vi "Key Scan Converter.vi"(5 "Input Scancode":i16, 6 "Input Key":string="nul") -> (1 "Scancode -> Key":string, 2 "Key -> Scancode":i16)   [LabVIEW 2017]
doc: "Converts back and forth between Keyboard Keys and Keyboard Decimal values. Automatically handles either Mac or PC. For ease of use with Event Structures."
panel:
  out "Scancodes":i32[](array[numeric])
  out "Keys":string[](array[string])
  in  "Scancode Table":string[][](array[string])=[["ID", "Key", "PC-HEX", "PC-DEC", "MAC-DEC", ""], ["1", "ESC", "1", "1", "53", ""], ["2", "1", "2", "2", "18", ""], ["3", "2", "3", "3", "19", ""], ["4", "3", "4", "4", "20", ""], ["5", "4", "5", "5", "21", ""], ["6", "5", "6", "6", "23", ""], ["7", "6", "7", "7", "22", ""], ["8", "7", "8", "8", "26", ""], ["9", "8", "9", "9", "28", ""], ["10", "9", "0A", "10", "25", ""], ["11", "0", "0B", "11", "29", ""], ["12", "-", "0C", "12", "27", ""], ["13", "=", "0D", "13", "24", ""], ["14", "BKSP", "0E", "14", "51", ""], ["15", "Tab", "0F", "15", "48", ""], ["16", "Q", "10", "16", "12", ""], ["17", "W", "11", "17", "13", ""], ["18", "E", "12", "18", "14", ""], ["19", "R", "13", "19", "15", ""], ["20", "T", "14", "20", "17", ""], ["21", "Y", "15", "21", "16", ""], ["22", "U", "16", "22", "32", ""], ["23", "I", "17", "23", "34", ""], ["24", "O", "18", "24", "31", ""], ["25", "P", "19", "25", "35", ""], ["26", "[", "1A", "26", "33", ""], ["27", "]", "1B", "27", "30", ""], ["28", "Enter", "1C", "28", "36", ""], ["29", "Ctrl", "1D", "29", "59", ""], ["30", "A", "1E", "30", "0", ""], ["31", "S", "1F", "31", "1", ""], ["32", "D", "20", "32", "2", ""], ["33", "F", "21", "33", "3", ""], ["34", "G", "22", "34", "5", ""], ["35", "H", "23", "35", "4", ""], ["36", "J", "24", "36", "38", ""], ["37", "K", "25", "37", "40", ""], ["38", "L", "26", "38", "37", ""], ["39", ";", "27", "39", "41", ""], ["40", "", "28", "40", "", ""], ["41", "`", "29", "41", "", ""], ["42", "L SH", "2A", "42", "", ""], ["43", "\\", "2B", "43", "", ""], ["44", "Z", "2C", "44", "6", ""], ["45", "X", "2D", "45", "7", ""], ["46", "C", "2E", "46", "8", ""], ["47", "V", "2F", "47", "9", ""], ["48", "B", "30", "48", "11", ""], ["49", "N", "31", "49", "45", ""], ["50", "M", "32", "50", "46", ""], ["51", "\"", "\"", "33", "51", ""], ["52", ".", "34", "52", "", ""], ["53", "/", "35", "53", "", ""], ["54", "R SH", "36", "54", "", ""], ["55", "PrintScreen", "37", "55", "", ""], ["56", "Alt", "38", "56", "", ""], ["57", "Space", "39", "57", "49", ""], ["58", "CpsLk", "3A", "58", "", ""], ["59", "F1", "3B", "59", "", ""], ["60", "F2", "3C", "60", "", ""], ["61", "F3", "3D", "61", "", ""], ["62", "F4", "3E", "62", "", ""], ["63", "F5", "3F", "63", "", ""], ["64", "F6", "40", "64", "", ""], ["65", "F7", "41", "65", "", ""], ["66", "F8", "42", "66", "", ""], ["67", "F9", "43", "67", "", ""], ["68", "F10", "44", "68", "", ""], ["69", "Num Lk", "45", "69", "", ""], ["70", "Scrl Lk", "46", "70", "", ""], ["71", "Home", "47", "71", "", ""], ["72", "Up Arrow", "48", "72", "126", ""], ["73", "Pg Up", "49", "73", "", ""], ["74", "- (num)", "4A", "74", "", ""], ["75", "Left Arrow", "4B", "75", "123", ""], ["76", "5 (num) ", "4C", "76", "", ""], ["77", "Right Arrow", "4D", "77", "124", ""], ["78", "+ (num)", "4E", "78", "", ""], ["79", "1 End", "4F", "79", "", ""], ["80", "Down Arrow", "50", "80", "125", ""], ["81", "3 Pg Dn", "51", "81", "", ""], ["82", "0 Ins", "52", "82", "", ""], ["83", "Del", "53", "83", "117", ""], ["84", "SH F1", "54", "84", "", ""], ["85", "SH F2", "55", "85", "", ""], ["86", "SH F3", "56", "86", "", ""], ["87", "SH F4", "57", "87", "", ""], ["88", "SH F5", "58", "88", "", ""], ["89", "SH F6", "59", "89", "", ""], ["90", "SH F7", "5A", "90", "", ""], ["91", "SH F8", "5B", "91", "", ""], ["92", "SH F9", "5C", "92", "", ""], ["93", "SH F10", "5D", "93", "", ""], ["94", "Ctrl F1", "5E", "94", "", ""], ["95", "Ctrl F2", "5F", "95", "", ""], ["96", "Ctrl F3", "60", "96", "", ""], ["97", "Ctrl F4", "61", "97", "", ""], ["98", "Ctrl F5", "62", "98", "", ""], ["99", "Ctrl F6", "63", "99", "", ""], ["100", "Ctrl F7", "64", "100", "", ""], ["101", "Ctrl F8", "65", "101", "", ""], ["102", "Ctrl F9", "66", "102", "", ""], ["103", "Ctrl F10", "67", "103", "", ""], ["104", "Alt F1", "68", "104", "", ""], ["105", "Alt F2", "69", "105", "", ""], ["106", "Alt F3", "6A", "106", "", ""], ["107", "Alt F4", "6B", "107", "", ""], ["108", "Alt F5", "6C", "108", "", ""], ["109", "Alt F6", "6D", "109", "", ""], ["110", "Alt F7", "6E", "110", "", ""], ["111", "Alt F8", "6F", "111", "", ""], ["112", "Alt F9", "70", "112", "", ""], ["113", "Alt F10", "71", "113", "", ""], ["114", "Ctrl PtScr", "72", "114", "", ""], ["115", "Ctrl L Arrow", "73", "115", "", ""], ["116", "Ctrl R Arrow", "74", "116", "", ""], ["117", "Ctrl End", "75", "117", "", ""], ["118", "Ctrl PgDn", "76", "118", "", ""], ["119", "Ctrl Home", "77", "119", "", ""], ["120", "Alt 1", "78", "120", "", ""], ["121", "Alt 2", "79", "121", "", ""], ["122", "Alt 3", "7A", "122", "", ""], ["123", "Alt 4", "7B", "123", "", ""], ["124", "Alt 5", "7C", "124", "", ""], ["125", "Alt 6", "7D", "125", "", ""], ["126", "Alt 7", "7E", "126", "", ""], ["127", "Alt 8", "7F", "127", "", ""], ["128", "Alt 9", "80", "128", "", ""], ["129", "Alt 0", "81", "129", "", ""], ["130", "Alt - ", "82", "130", "", ""], ["131", "Alt =", "82", "130", "", ""], ["132", "Ctrl PgUp", "84", "132", "", ""], ["133", "F11", "85", "133", "", ""], ["134", "F12", "86", "134", "", ""], ["135", "SH F11", "87", "135", "", ""], ["136", "SH F12", "88", "136", "", ""], ["137", "Ctrl F11", "89", "137", "", ""], ["138", "Ctrl F12", "8A", "138", "", ""], ["139", "Alt F11", "8B", "139", "", ""], ["140", "Alt F12", "8C", "140", "", ""], ["141", "Ctrl Up Arrow", "8C", "140", "", ""], ["142", "Ctrl - (num)", "8E", "142", "", ""], ["143", "Ctrl 5 (num)", "8F", "143", "", ""], ["144", "Ctrl + (num)", "90", "144", "", ""], ["145", "Ctrl Dn  Arrow", "91", "145", "", ""], ["146", "Ctrl Ins", "92", "146", "", ""], ["147", "Ctrl Del", "93", "147", "", ""], ["148", "Ctrl Tab", "94", "148", "", ""], ["149", "Ctrl / (num)", "95", "149", "", ""], ["150", "Ctrl * (num)", "96", "150", "", ""], ["151", "Alt Home", "97", "151", "", ""], ["152", "Alt Up Arrow", "98", "152", "", ""], ["153", "Alt PgUp", "99", "153", "", ""], ["154", "", "9A", "154", "", ""], ["155", "Alt Left Arrow", "9B", "155", "", ""], ["156", "", "9C", "156", "", ""], ["157", "Alt Rt Arrow", "9D", "157", "", ""], ["158", "", "9E", "158", "", ""], ["159", "Alt End", "9F", "159", "", ""], ["160", "Alt Dn Arrow", "A0", "160", "", ""], ["161", "Alt PgDn", "A1", "161", "", ""], ["162", "Alt Ins", "A2", "162", "", ""], ["163", "Alt Del", "A3", "163", "", ""], ["164", "Alt / (num)", "A4", "164", "", ""], ["165", "Alt Tab", "A5", "165", "", ""], ["166", "Alt Enter (num)", "A6", "166", "", ""]]
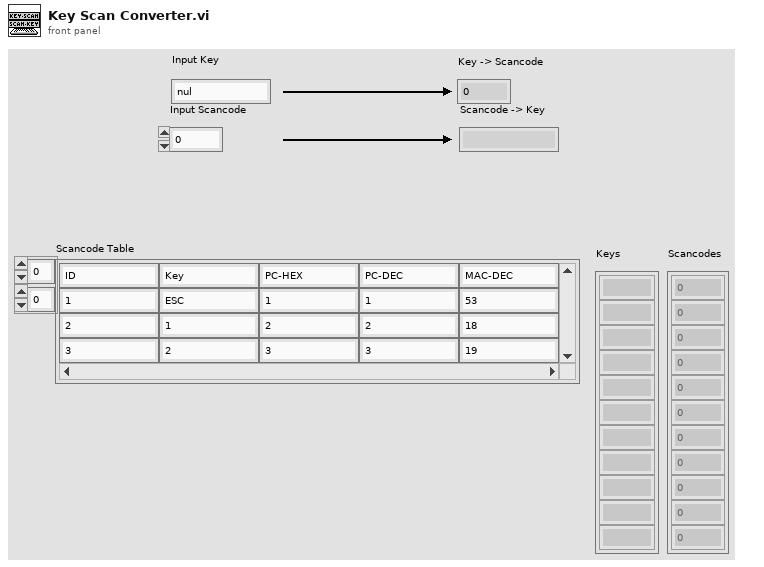
[diagram p1: front panel]
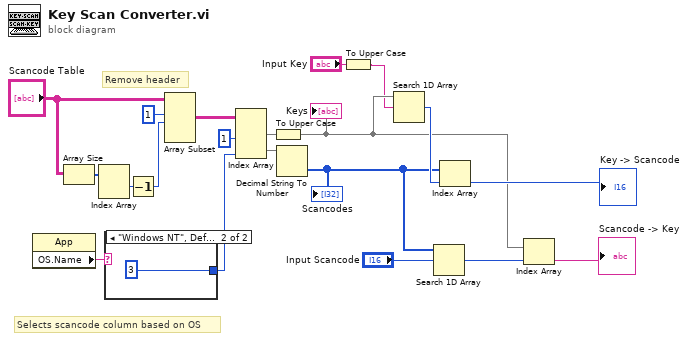
[diagram p0: block diagram]
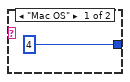
[diagram p2: hidden frame]
diagram:
  # "Selects scancode column based on OS"
  # "Remove header"
  n1 = property class="App"() -> ("OS.Name"=w7:string)  [unwired: 2 in, 2 out]
  n2 = Array Size(array="Scancode Table") -> (size(s)=w18:i32[])
  n3 = Index Array(array=w18) -> (element #1=w15:i32)  [unwired: 2 in, 1 out]
  n4 = case shown="\"Windows NT\", Default" w7 {
    tunnel: [4 ("index (col)") 3 ("index (col)")] -> w5
    frame "Mac OS" {
    }
    frame "Windows NT", Default {
    }
  }
  n5 = Decrement(x=w15) -> (x-1=w16:i32)
  n6 = Array Subset(array="Scancode Table", index (row)=1 ("index"), length (row)=w16) -> (w19:string[][])  [unwired: 2 in]
  n7 = Index Array(array=w19, index (col) #1=1 ("disabled index (col)"), index (col) #2=w5) -> (element #1=w3:string[], element #2=w14:string[])  [unwired: 2 in]
  n8 = To Upper Case(1:w3) -> (0:w4:string[])
  "Keys" <- w4
  n9 = Decimal String To Number(string=w14) -> (number=w9:i32[])  [unwired: 2 in, 1 out]
  "Scancodes" <- w9
  n10 = To Upper Case(1:"Input Key") -> (0:w1:string)
  n11 = Search 1D Array(1D array=w4, element=w1) -> (index of element=w10:i32)  [unwired: 1 in]
  n12 = Search 1D Array(1D array=w9, element="Input Scancode") -> (index of element=w12:i32)  [unwired: 1 in]
  n13 = Index Array(array=w9, index=w10) -> (element=→"Key -> Scancode":i32)
  n14 = Index Array(array=w4, index=w12) -> (element=→"Scancode -> Key":string)
